vi "Update Value.vi"(6 "Time":dbl, 8 "error in (no error)":errorcluster, 11 "LocalGraphBuffer in":refnum<class "LocalGraphBuffer.lvclass">) -> (0 "error out":errorcluster, 1 "Update":bool, 2 "Value":variant, 3 "LocalGraphBuffer out":refnum<class "LocalGraphBuffer.lvclass">)   [LabVIEW 2020, in "VolatusGUIElements.lvlib" / "LocalGraphBuffer.lvclass"]
uses:
  LocalGraphBuffer.lvclass
  LocalGraphBuffer.lvclass/LocalGraphBuffer.ctl
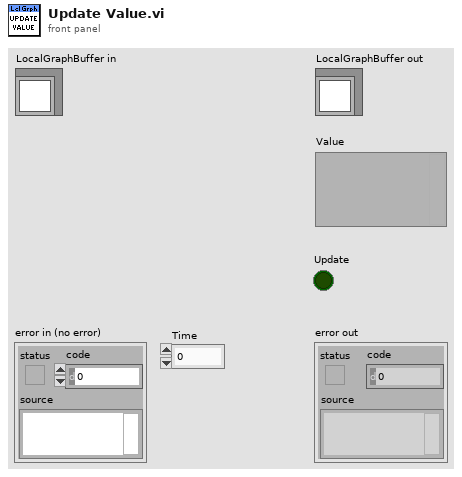
[diagram p1: front panel]
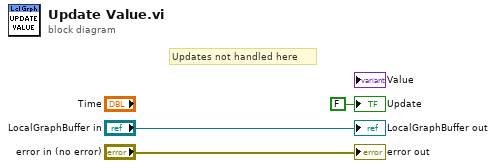
[diagram p0: block diagram]
diagram:
  # "Updates not handled here"
  "error out" <- "error in (no error)"
  "LocalGraphBuffer out" <- "LocalGraphBuffer in"
  "Update" <- FALSE ("Update")
